vi "Circle detection.vi"() -> ()   [LabVIEW 2014]
uses:
  Resources/Global.vi
  <vilib>/vision/NI_Vision_Development_Module.lvlib
  <vilib>/LVH/AR Drone Toolkit/Decode Video/2.0/Decode20Video.dll
panel:
  in  "Circle Index":i32
  out "Number of Matches Returned":i32
  out "error out":errorcluster
  out "Image":T1(plugin-control)
  in  "milliseconds to wait":u32
  out "x-y":u32=19
  # "Do NOT un this VI. Instead run \"AR.Drone MAIN.vi\" and select the name of this VI in the dop-down menu at the Steup tab"
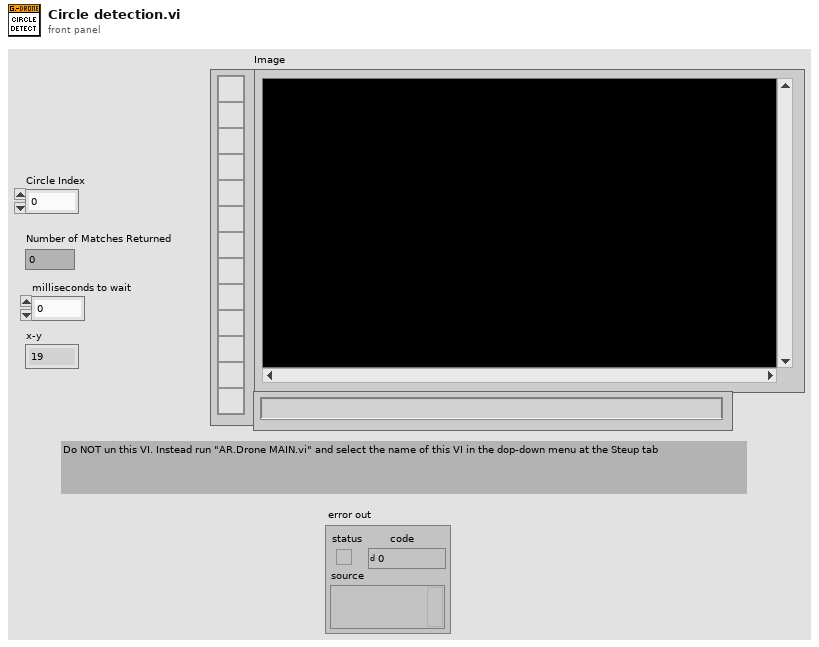
[diagram p1: front panel]
types:
  T1 = typedef "IMAQ Image.ctl" = refnum<image>
  T2 = typedef "Image Type" = u32
  T3 = cluster{"Position":cluster{"X":sgl, "Y":sgl}, "Radius":dbl, "Score":dbl}[]
  T4 = cluster{"Position":cluster{"X":sgl, "Y":sgl}, "Radius":dbl, "Score":dbl}
  T5 = cluster{"Left":i32, "Top":i32, "Right":i32, "Bottom":i32}
  T6 = typedef "Control cluster.ctl" = cluster{"Roll":sgl, "Pitch":sgl, "Vertical Speed":sgl, "Yaw Speed":sgl}
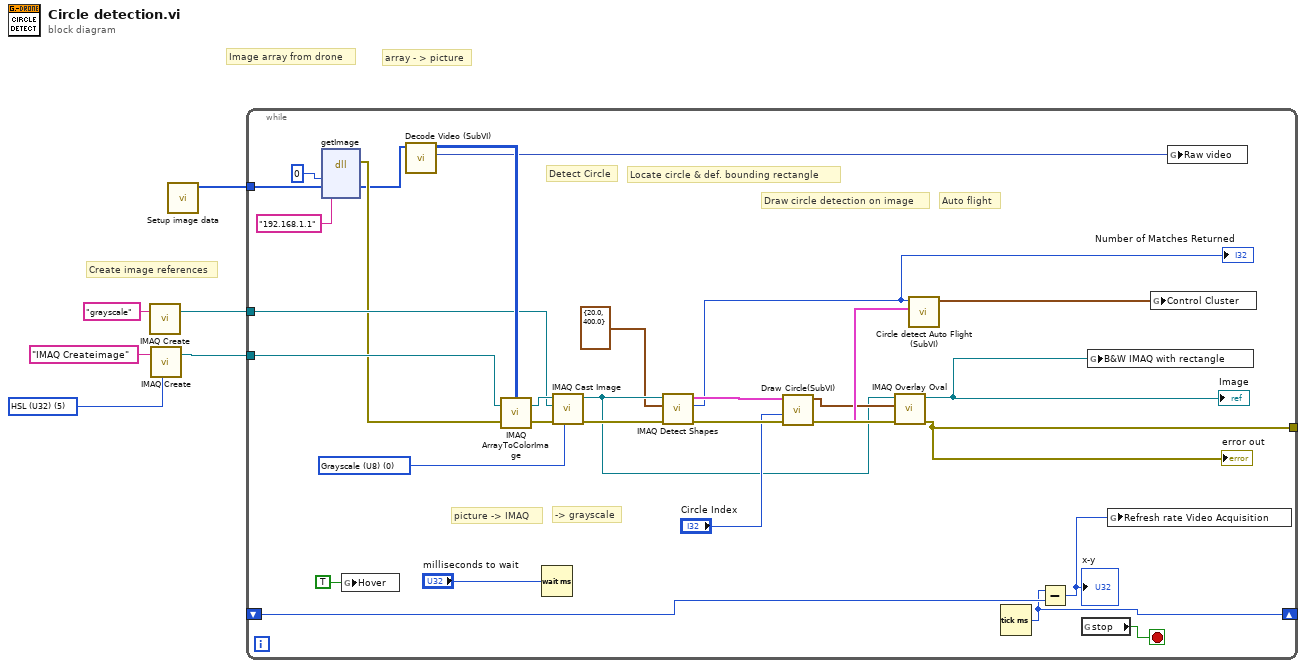
[diagram p0: block diagram]
diagram:
  w4 = T2 5 items=["Grayscale (U8)", "Grayscale (I16)", "Grayscale (SGL)", "Complex (CSG)", "RGB (U32)", "HSL (U32)", "RGB (U64)", "Grayscale (U16)"] ("Image Type")
  # "Create image references"
  # "array - > picture"
  # "Image array from drone"
  n1 = call "IMAQ Create"("Image Name"="grayscale") -> ("New Image"=w3:T1)  [unwired: 4 in, 1 out]
  n2 = call "IMAQ Create"("Image Name"="IMAQ Createimage", "Image Type"=w4) -> ("New Image"=w5:T1)  [unwired: 3 in, 1 out]
  n3 = call "Setup image data.vi"() -> ("Array"=w1:u8[])  [unwired: 11 in]
  n4 = while {
    shift-right: [w8] -> _
    shift-left: _ -> [w34]
    tunnel: w5 -> [w20]
    tunnel: w3 -> [w19]
    tunnel: w1 -> [w10]
    tunnel: [w15] -> _
    stop <- w22 stop-if-true
    w31 = T2 0 items=["Grayscale (U8)", "Grayscale (I16)", "Grayscale (SGL)", "Complex (CSG)", "RGB (U32)", "HSL (U32)", "RGB (U64)", "Grayscale (U16)"] ("Image Type")
    # "-> grayscale"
    # "picture -> IMAQ"
    # "Auto flight"
    # "Draw circle detection on image"
    # "Locate circle & def. bounding rectangle"
    # "Detect Circle"
    n5 = dll-call lib="C:/Program Files (x86)/National Instruments/LabVIEW 2014/vi.lib/LVH/AR Drone Toolkit/Decode Video/2.0/Decode20Video.dll" fn="getImage"("Index"=0, "ImgData"=w10, "IP Address"="192.168.1.1") -> (error out=w13:errorcluster, "ImgData"=w12:u8[])  [unwired: 6 in, 1 out]
    n6 = global write "Global.vi" "Hover"(TRUE) -> ()
    n7 = call "Decode Video (SubVI).vi"("ImgData"=w12) -> ("new picture"=w33:picture, "Array"=w35:u32[][])  [unwired: 9 in]
    n8 = call "IMAQ ArrayToColorImage"("Image Pixels (U32)"=w35, "Image"=w20, "error in (no error)"=w13) -> ("Image Out"=w32:T1, "error out"=w21:errorcluster)  [unwired: 2 in]
    n9 = Wait (ms)(milliseconds to wait="milliseconds to wait") -> ()  [unwired: 1 out]
    n10 = call "IMAQ Cast Image"("Image Type"=w31, "error in (no error)"=w21, "Image Dst"=w19, "Image Src"=w32) -> ("error out"=w30:errorcluster, "Image Dst Out"=w17:T1)  [unwired: 6 in]
    n11 = call-poly "IMAQ Detect Shapes"("error in (no error)"=w30, "Circle Descriptor"=cluster{"Min Radius":dbl, "Max Radius":dbl} {"Min Radius"=20.0, "Max Radius"=400.0}, "Image"=w17) -> ("error out"=w29:errorcluster, "Number of Matches Returned"=w16:i32, "Circles"=w28:T3)  [unwired: 6 in]
    "Number of Matches Returned" <- w16
    n12 = call "Draw Circle(SubVI).vi"("Circle Index"="Circle Index", "Circles"=w28) -> ("element"=w27:T4, "Bounding Rectangle out"=w18:T5)  [unwired: 7 in, 1 out]
    n13 = call "IMAQ Overlay Oval"("error in (no error)"=w29, "Bounding Rectangle"=w18, "Image"=w17) -> ("error out"=w15:errorcluster, "Image Out"=w25:T1)  [unwired: 7 in]
    "Image" <- w25
    "error out" <- w15
    n14 = call "Circle detect Auto Flight (SubVI).vi"("element"=w27, "Number of Matches Returned"=w16) -> ("Control Cluster out"=w26:T6)  [unwired: 9 in]
    n15 = Tick Count (ms)() -> (millisecond timer value=w8:u32)
    n16 = Subtract(x=w8, y=w34) -> (x-y=w7:u32)
    "x-y" <- w7
    n17 = global read "Global.vi" "stop"() -> (w22:bool)
    n18 = global write "Global.vi" "B&W IMAQ with rectangle"(w25) -> ()
    n19 = global write "Global.vi" "Refresh rate Video Acquisition"(w7) -> ()
    n20 = global write "Global.vi" "Control Cluster"(w26) -> ()
    n21 = global write "Global.vi" "Raw video"(w33) -> ()
  }
